vi "CSV_WhileLoop_Iter.vi"() -> ()   [LabVIEW 2021]
uses:
  <vilib>/DAQmx/write.llb/DAQmx Write (Analog 1D DBL NChan 1Samp).vi
  <vilib>/DAQmx/create/channels.llb/DAQmx Create Channel (AO-Voltage-Basic).vi
  <vilib>/Utility/file.llb/Read Delimited Spreadsheet (I64).vi
  <vilib>/DAQmx/configure/timing.llb/DAQmx Timing (Sample Clock).vi
  <vilib>/DAQmx/miscellaneous.llb/DAQmx Fill In Error Info.vi
panel:
  out "Phase II Iterations 2":i32
  out "Phase II Iterations":i32
  in  "TickLength":u32
  in  "Y1 (-10-10V)":dbl
  in  "X1 (-10-10V)":dbl
  in  "Blanking (0-10v)":dbl=10.0
  in  "514 (0-10v)":dbl
  in  "488 (0-10v)":dbl
  in  "445 (0-10v)":dbl
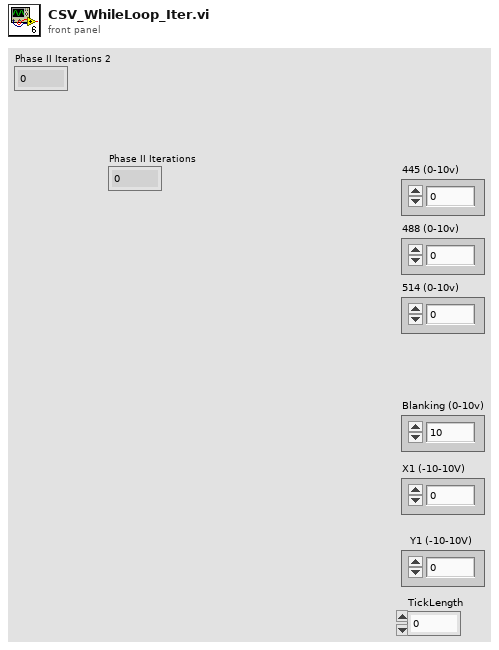
[diagram p1: front panel]
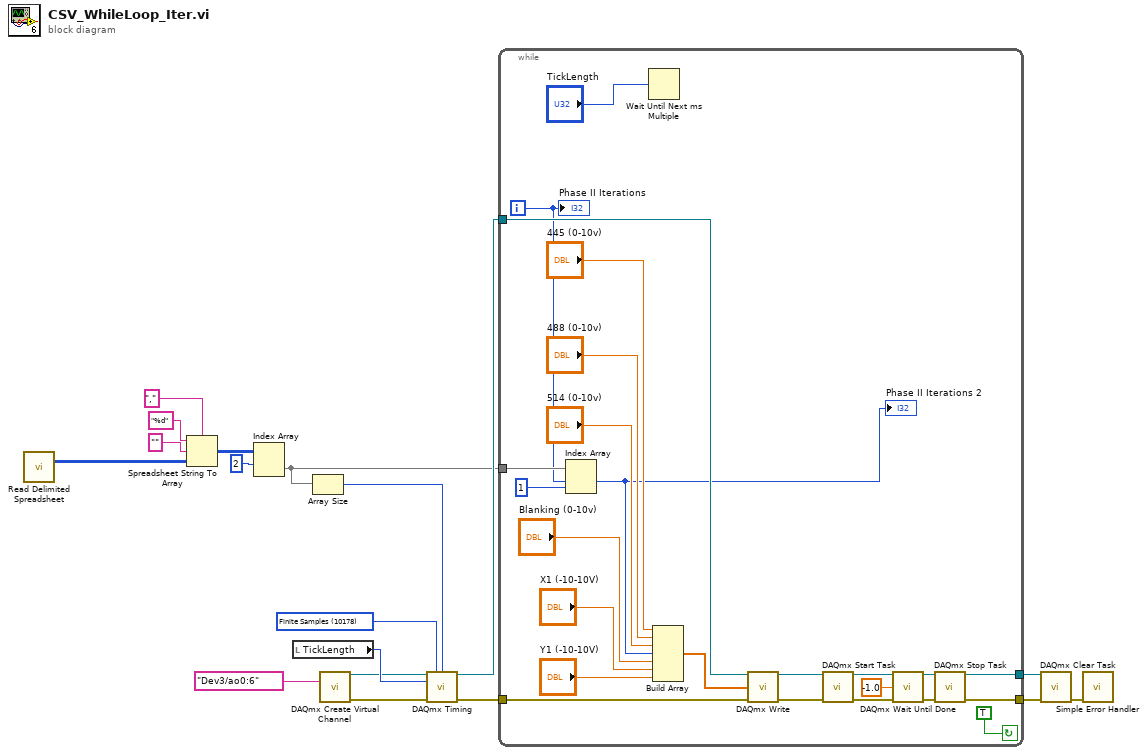
[diagram p0: block diagram]
diagram:
  w11 = 10178 items=["Finite Samples"=10178, "Continuous Samples"=10123, "Hardware Timed Single Point"=12522] ("sample mode")
  n1 = call-poly <vilib>:"Read Delimited Spreadsheet.vi"() -> ("all rows"=w16:i64[][])  [unwired: 10 in, 5 out]
  n2 = Spreadsheet String To Array(delimiter (Tab)=",", format string="%d", spreadsheet string="", array type (2D Dbl)=w16) -> (array=w1:i64[][])
  n3 = Index Array(array=w1, index (row)=2) -> (element=w2:i64[])  [unwired: 1 in]
  n4 = local read "TickLength"() -> (w10:u32)
  n5 = Array Size(array=w2) -> (size(s)=w7:i32)
  n6 = call-poly <vilib>:"DAQmx Create Virtual Channel.vi"("physical channels"=tag "Dev3/ao0:6") -> ("task out"=w6:refnum<k21>, "error out"=w5:errorcluster)  [unwired: 13 in]
  n7 = call-poly <vilib>:"DAQmx Timing.vi"("task/channels in"=w6, "sample mode"=w11, "samples per channel"=w7, "rate"=w10, "error in"=w5) -> ("task out"=w3:refnum<k21>, "error out"=w4:errorcluster)  [unwired: 9 in]
  n8 = while {
    tunnel: [w28] -> w9
    tunnel: [w29] -> w8
    tunnel: w4 -> [w24]
    tunnel: w3 -> [w23]
    tunnel: w2 -> [w22]
    i -> [w21]
    stop <- TRUE continue-if-true
    n9 = Index Array "Index Array"(array=w22, index #1=w21, index #2=1) -> (element #1=w19:i64)  [unwired: 1 out]
    "Phase II Iterations 2" <- w19
    n10 = Wait Until Next ms Multiple(millisecond multiple="TickLength") -> ()  [unwired: 1 out]
    n11 = Build Array("445 (0-10v)", "488 (0-10v)", "514 (0-10v)", w19, "Blanking (0-10v)", "X1 (-10-10V)", "Y1 (-10-10V)") -> (w42:dbl[])
    n12 = call-poly <vilib>:"DAQmx Write.vi"("task/channels in"=w23, "data"=w42, "error in"=w24) -> ("task out"=w25:refnum<k21>, "error out"=w32:errorcluster)  [unwired: 10 in, 1 out]
    n13 = call <vilib>:"DAQmx Start Task.vi"("task/channels in"=w25, "error in"=w32) -> ("task out"=w26:refnum<k21>, "error out"=w31:errorcluster)  [unwired: 12 in]
    n14 = call <vilib>:"DAQmx Wait Until Done.vi"("task/channels in"=w26, "timeout (sec)"=-1.0, "error in"=w31) -> ("task out"=w27:refnum<k21>, "error out"=w30:errorcluster)  [unwired: 11 in]
    n15 = call <vilib>:"DAQmx Stop Task.vi"("task/channels in"=w27, "error in"=w30) -> ("task out"=w28:refnum<k21>, "error out"=w29:errorcluster)  [unwired: 12 in]
    "Phase II Iterations" <- w21
  }
  n16 = call <vilib>:"DAQmx Clear Task.vi"("task in"=w9, "error in"=w8) -> ("error out"=w18:errorcluster)  [unwired: 13 in]
  n17 = call <vilib>:"Simple Error Handler.vi"("error in (no error)"=w18) -> ()  [unwired: 4 in, 5 out]
